vi "客户机.vi"() -> ()   [LabVIEW 2017]
panel:
  out "波形图":dbl[](graph)
  in  "x":i32(slide) scale=0.0..10.0
  in  "停止":bool
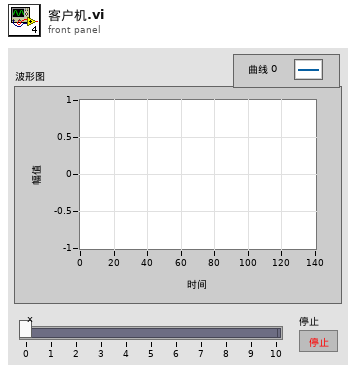
[diagram p1: front panel]
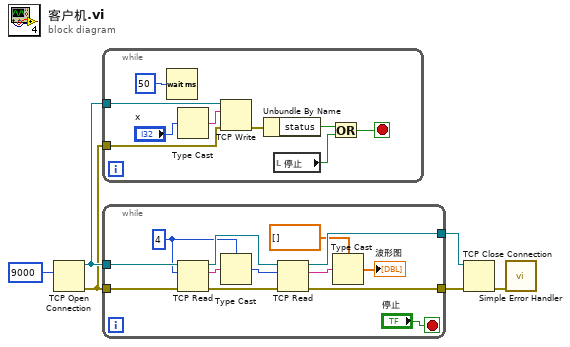
[diagram p0: block diagram]
diagram:
  n1 = TCP Open Connection(remote port or service name=u16 9000 ("远程端口或服务名称")) -> (connection ID=w3:refnum<k5>, error out=w2:errorcluster)  [unwired: 4 in]
  n2 = while {
    tunnel: w3 -> [w15]
    tunnel: w2 -> [w13]
    stop <- w10 stop-if-true
    n3 = Wait (ms)(milliseconds to wait=u32 50 ("等待时间（毫秒）")) -> ()  [unwired: 1 out]
    n4 = Type Cast(x="x") -> (*(type *) &x=w14:string)  [unwired: 1 in]
    n5 = TCP Write(connection ID=w15, data in=w14, error in (no error)=w13) -> (error out=w9:errorcluster)  [unwired: 1 in, 2 out]
    n6 = Unbundle By Name(w9) -> ("status"=w12:bool)
    n7 = local read "停止"() -> (w11:bool)
    n8 = Or(x=w12, y=w11) -> (x .or. y?=w10:bool)
  }
  n9 = while {
    tunnel: w3 -> [w27]
    tunnel: w2 -> [w26]
    tunnel: [w23] -> w6
    tunnel: [w22] -> w5
    stop <- "停止" stop-if-true
    w20 = 4
    n10 = TCP Read(connection ID=w27, bytes to read=w20, error in (no error)=w26) -> (connection ID out=w25:refnum<k5>, data out=w21:string, error out=w24:errorcluster)  [unwired: 2 in]
    n11 = Type Cast(type=w20, x=w21) -> (*(type *) &x=w19:i32)
    n12 = TCP Read(connection ID=w25, bytes to read=w19, error in (no error)=w24) -> (connection ID out=w23:refnum<k5>, data out=w18:string, error out=w22:errorcluster)  [unwired: 2 in]
    n13 = Type Cast(type=dbl[] [] ("Sinusoidal Pattern"), x=w18) -> (*(type *) &x=→"波形图":dbl[])
  }
  n14 = TCP Close Connection(connection ID=w6, error in (no error)=w5) -> (error out=w1:errorcluster)  [unwired: 1 in, 1 out]
  n15 = call <vilib>:"Simple Error Handler.vi"("error in (no error)"=w1) -> ()  [unwired: 4 in, 5 out]
